vi "Receive CCD Status.vi"(8 "error in (no error)":errorcluster, 11 "Stream in":refnum<class "Stream.lvclass">) -> (0 "error out":errorcluster, 3 "Stream out":refnum<class "Stream.lvclass">)   [LabVIEW 2018, in "Stream.lvclass"]
uses:
  Stream.lvclass
  Interface/Interface.lvclass
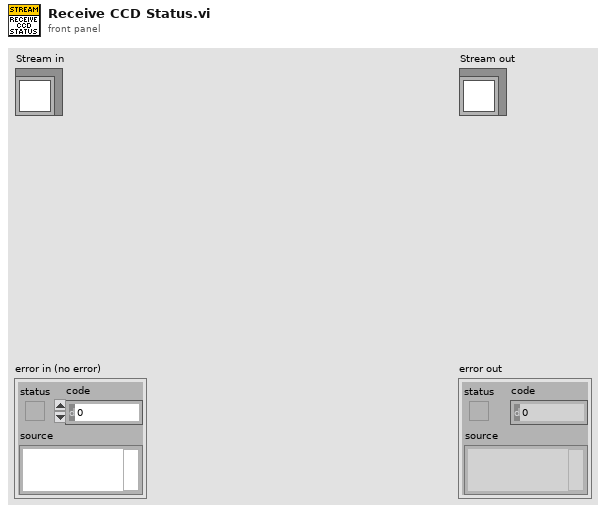
[diagram p1: front panel]
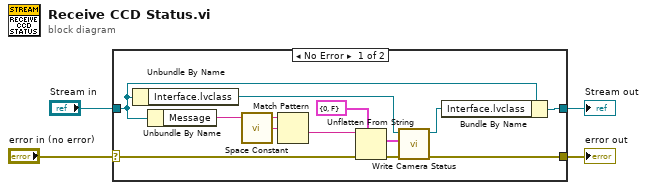
[diagram p0: block diagram]
diagram:
  n1 = case shown="No Error" "error in (no error)" {
    selector: "error in (no error)" -> [w13 w18]
    tunnel: [w12 w18] -> w3
    tunnel: [w10 w17] -> w1
    tunnel: "Stream in" -> [w11 w17]
    frame No Error {
      n2 = Unbundle By Name(w11) -> ("Interface.lvclass"=w9:refnum<class "Interface.lvclass">)
      n3 = Unbundle By Name(w11) -> ("Message"=w16:string)
      n4 = call <vilib>:"Space Constant.vi"() -> ("String"=w15:string)
      n5 = Match Pattern(string=w16, regular expression=w15) -> (after substring=w14:string)  [unwired: 1 in, 3 out]
      n6 = Unflatten From String(type=cluster{"% Acquired":u16, "Acquiring":bool} {"% Acquired"=0, "Acquiring"=FALSE} ("Camera Status"), binary string=w14, error in (no error)=w13) -> (value=w5:cluster{"% Acquired":u16, "Acquiring":bool}, error out=w7:errorcluster)  [unwired: 2 in, 1 out]
      n7 = call "Write Camera Status.vi"("error in (no error)"=w7, "Camera Status"=w5, "Interface in"=w9) -> ("error out"=w12:errorcluster, "Interface out"=w8:refnum<class "Interface.lvclass">)  [unwired: 7 in]
      n8 = Bundle By Name(cluster=w11, "Interface.lvclass"=w8) -> (w10:refnum<class "Stream.lvclass">)
    }
    frame Error {
    }
  }
  "error out" <- w3
  "Stream out" <- w1
